vi "Write Amt_fb_user Msg.vi"(9 "Root Controller":refnum<class "Message Enqueuer.lvclass">, 10 "Database_handler.lvlib:Amt_fb_user Msg.lvclass":refnum<class "Amt_fb_user Msg.lvclass">, 11 "Database_handler in":refnum<class "Database_handler.lvclass">) -> (3 "Database_handler out":refnum<class "Database_handler.lvclass">)   [LabVIEW 2025, in "Database_handler.lvlib" / "Database_handler.lvclass"]
uses:
  Database_handler.lvclass
  Database_handler Messages/Amt_fb_user Msg/Amt_fb_user Msg.lvclass
  Database_handler.lvclass/Database_handler.ctl
  <vilib>/ActorFramework/Message Enqueuer/Message Enqueuer.lvclass
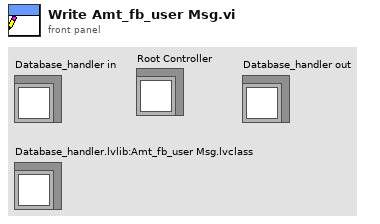
[diagram p1: front panel]
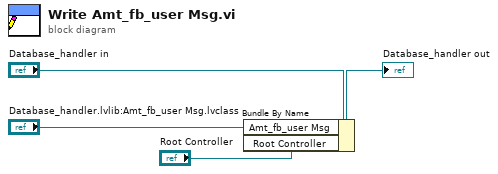
[diagram p0: block diagram]
diagram:
  n1 = Bundle By Name(cluster="Database_handler in", "Amt_fb_user Msg"="Database_handler.lvlib:Amt_fb_user Msg.lvclass", "Root Controller"="Root Controller") -> (→"Database_handler out":refnum<class "Database_handler.lvclass">)
